vi "InitFromXML.vi"(8 "error in (no error)":errorcluster, 10 "XML":string, 11 "RingItem in":refnum<class "RingItem.lvclass">) -> (0 "error out":errorcluster, 3 "RingItem out":refnum<class "RingItem.lvclass">)   [LabVIEW 2009, in "NavScreen.lvlib" / "RingItem.lvclass"]
uses:
  RingItem.lvclass
  Link/Link.lvclass
  RingItem.lvclass/RingItem.ctl
  NavScreen.lvlib
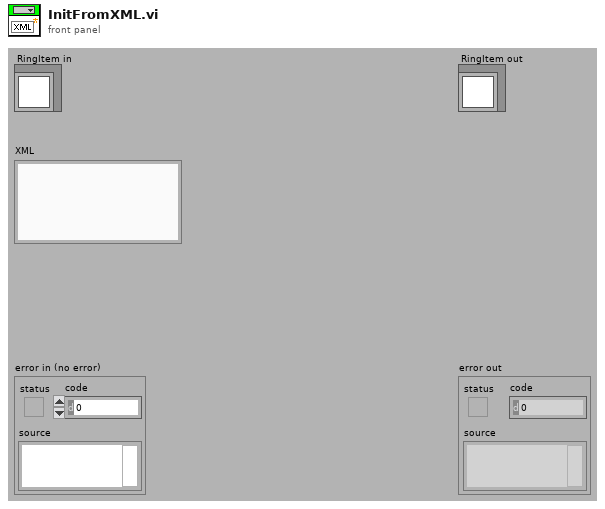
[diagram p1: front panel]
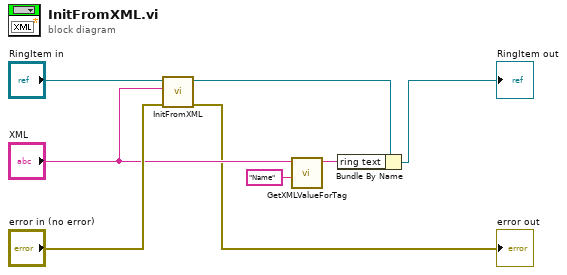
[diagram p0: block diagram]
diagram:
  n1 = call-parent "InitFromXML.vi"("error in (no error)"="error in (no error)", "XML"="XML", "Link in"="RingItem in") -> ("error out"=→"error out":errorcluster, "Link out"=w4:refnum<class "RingItem.lvclass">)  [unwired: 7 in]
  n2 = call "GetXMLValueForTag.vi"("tag"="Name", "XML"="XML") -> ("value"=w7:string)  [unwired: 8 in, 1 out]
  n3 = Bundle By Name(cluster=w4, "ring text"=w7) -> (→"RingItem out":refnum<class "RingItem.lvclass">)
